vi "StartGui.vi"(0 "reference in":refnum<class "RemoteControl.lvclass">, 3 "ms timeout (-1)":i32=-1, 5 "error in (no error)":errorcluster) -> (14 "reference out":refnum<class "RemoteControl.lvclass">, 15 "EventFromProcess":refnum<user-event>, 16 "timed out":bool, 19 "error out":errorcluster)   [LabVIEW 2020, in "RemoteControl.lvclass"]
doc: "Looks up an existing object matching object name or creates a new object and returns a refnum you can use when calling other class methods.\n\nObjects created with this VI should be destroyed using this class Delete VI."
uses:
  RemoteControl.lvclass
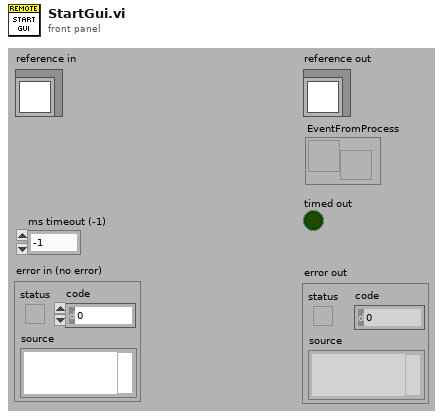
[diagram p1: front panel]
types:
  T1 = enum16{"ReadRepository", "CreateNew", "CreateOrLookUpExisting"}
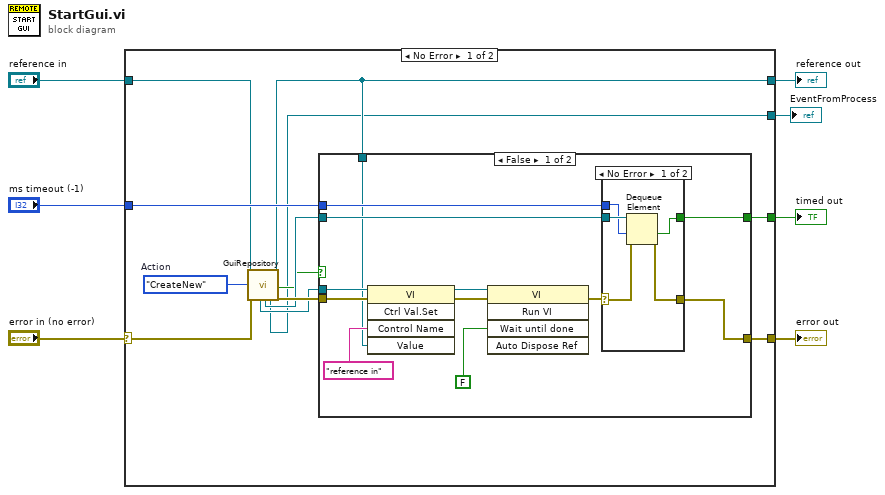
[diagram p0: block diagram]
diagram:
  n1 = case shown="No Error" "error in (no error)" {
    selector: "error in (no error)" -> [w15 w39]
    tunnel: [w17 w39] -> w6
    tunnel: [w11 w40] -> w4
    tunnel: "reference in" -> [w9 w40]
    tunnel: "ms timeout (-1)" -> [w19 _]
    tunnel: [w18 _] -> w2
    tunnel: [w8 _] -> w1
    frame No Error {
      w16 = T1."CreateNew"  # Action
      n2 = call "GuiRepository.vi"("reference in"=w9, "Action(ReadRepository)"=w16, "error in (no error)"=w15) -> ("ProcessViRef"=w13:refnum<vi>, "ProcessSyncQueue"=w12:refnum<queue>, "EventFromProcess"=w8:refnum<user-event>, "reference out"=w11:refnum<class "RemoteControl.lvclass">, "ProcessAlreadyStarted"=w10:bool, "error out"=w14:errorcluster)  [unwired: 9 in, 2 out]
      n3 = case shown="False" w10 {
        tunnel: w19 -> [w27 _]
        tunnel: [w26 _] -> w18
        tunnel: [w24 w38] -> w17
        tunnel: w14 -> [w23 w38]
        tunnel: w13 -> [w22 _]
        tunnel: w12 -> [w21 _]
        tunnel: w11 -> [w20 _]
        frame False {
          n4 = invoke class="VI" method="Ctrl Val.Set"(reference=w22, error in=w23, "Control Name"="reference in", "Value"=w20) -> (reference out=w30:refnum<vi>, error out=w29:errorcluster)  [unwired: 1 in, 3 out]
          n5 = invoke class="VI" method="Run VI"(reference=w30, error in=w29, "Wait until done"=FALSE ("Wait Until Done")) -> (error out=w25:errorcluster)  [unwired: 2 in, 4 out]
          n6 = case shown="No Error" w25 {
            tunnel: w21 -> [w36 _]
            tunnel: w27 -> [w34 _]
            tunnel: [w35 _] -> w26
            selector: w25 -> [w33 w37]
            tunnel: [w32 w37] -> w24
            frame No Error {
              n7 = Dequeue Element(queue=w36, timeout in ms (-1)=w34, error in (no error)=w33) -> (timed out?=w35:bool, error out=w32:errorcluster)  [unwired: 2 out]
            }
            frame Error {
            }
          }
        }
        frame True {
          # "Process Already started.\nThis option will only be used togeather with the\naction: \"CreateOrLookUpExisting\""
        }
      }
    }
    frame Error {
    }
  }
  "error out" <- w6
  "reference out" <- w4
  "timed out" <- w2
  "EventFromProcess" <- w1
